vi "Search Array.vi"(10 "element":string, 11 "array":string[](array[string])) -> (3 "indexes":i32[](array[numeric]))   [LabVIEW 2025]
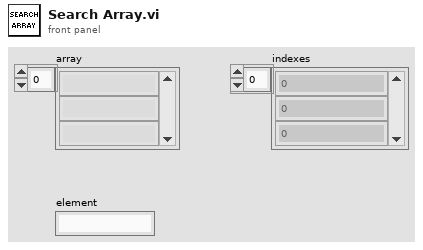
[diagram p1: front panel]
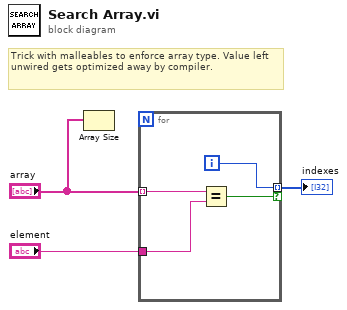
[diagram p0: block diagram]
diagram:
  # "Trick with malleables to enforce array type. Value left unwired gets optimized away by compiler."
  n1 = Array Size(array="array") -> ()  [unwired: 1 out]
  n2 = for {
    tunnel: "array" -> [w7] mode=indexing
    tunnel: "element" -> [w6]
    tunnel: [w5] -> w3 mode=indexing if=w4
    i -> [w5]
    n3 = Equal?(x=w7, y=w6) -> (x = y?=w4:bool)
  }
  "indexes" <- w3
